vi "Firing.vi"(9 "Off":bool, 10 "On":bool, 11 "Speed":dbl) -> (0 "error out":errorcluster, 3 "Is on":bool)   [LabVIEW 2012]
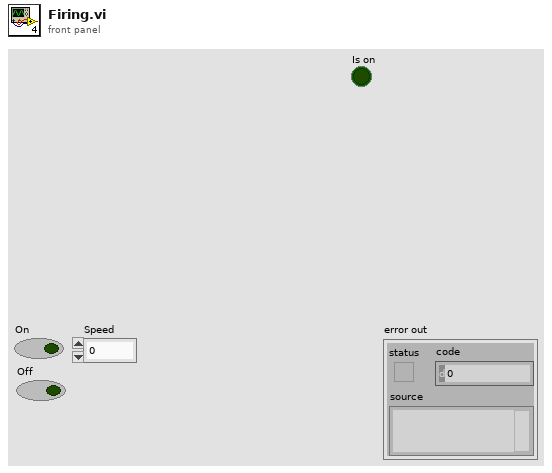
[diagram p1: front panel]
types:
  T1 = typedef "WPI_MotorControlDeviceRef.ctl" = cluster{"DeviceStatus":errorcluster, "Type":enum16{"PWM", "CAN"}, "PWM":cluster{"Digital Module":T2, "PWM Channel":T3, "DeadBand":T4}, "CAN":cluster{"Device Number":u8, "Control Mode":T5, "Semaphore":T6, "Max Vout":dbl}, "Invert":bool, "TransformRef":T7, "InvTransformRef":T7}
  T2 = typedef "FPGA_TypedefDigitalModule.ctl" = enum16{"Digital Module 1", "Digital Module 2"}
  T3 = typedef "FPGA_DIOPWMChannel.ctl" = enum8{"PWM 1", "PWM 2", "PWM 3", "PWM 4", "PWM 5", "PWM 6", "PWM 7", "PWM 8", "PWM 9", "PWM 10", "Invalid"}
  T4 = typedef "WPI_PWMDeadband.ctl" = cluster{"Name":string, "maxPositivePwm":i32, "minPositivePwm":i32, "centerPwm":i32, "maxNegativePwm":i32, "minNegativePwm":i32, "angularRange":u16}
  T5 = typedef "WPI_CANJaguar_ControlMode.ctl" = enum8{"Percent VBus", "Current", "Speed", "Position", "Voltage"}
  T6 = typedef "Semaphore RefNum" = refnum<k1>
  T7 = typedef "WPI_PWMTransform_ConPane.ctl" = refnum<vi>
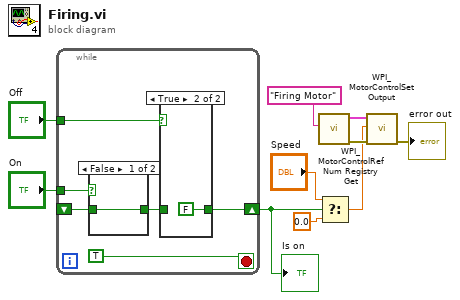
[diagram p0: block diagram]
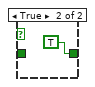
[diagram p2: hidden frame]
diagram:
  n1 = while {
    tunnel: "On" -> [w15]
    tunnel: "Off" -> [w14]
    shift-right: [w12] -> w4
    shift-left: _ -> [w11]
    stop <- TRUE stop-if-true
    n2 = case shown="False" w15 {
      tunnel: [w17 TRUE] -> w13
      tunnel: w11 -> [w17 _]
      frame False {
      }
      frame True {
      }
    }
    n3 = case shown="True" w14 {
      tunnel: [w19 FALSE] -> w12
      tunnel: w13 -> [w19 _]
      frame False {
      }
      frame True {
      }
    }
  }
  "Is on" <- w4
  n4 = call <vilib>:"WPI_MotorControlRefNum Registry Get.vi"("refnum name"="Firing Motor") -> ("error out"=w7:errorcluster, "MotorControlDevRef"=w6:T1)  [unwired: 9 in]
  n5 = Select(t="Speed", s=w4, f=0.0) -> (s? t:f=w1:dbl)
  n6 = call <vilib>:"WPI_MotorControlSetOutput.vi"("error in (no error)"=w7, "Output"=w1, "MotorControlDevRef"=w6) -> ("error out"=→"error out":errorcluster)  [unwired: 6 in, 2 out]
